vi "Kinect test.vi"() -> ()   [LabVIEW 2017]
uses:
  <vilib>/MakerHub/KinectOne/Private/Type Defs/HandLeftState.ctl
  <vilib>/MakerHub/KinectOne/Private/Initialize Image [Body Index].vi
  <vilib>/MakerHub/KinectOne/Private/Initialize Image [Depth].vi
  <vilib>/MakerHub/KinectOne/Private/Initialize Image [Color].vi
  <vilib>/MakerHub/KinectOne/Private/kinectRead [BodyIndexFrame].vi
  <vilib>/MakerHub/KinectOne/Private/kinectRead [DepthFrame].vi
  <vilib>/MakerHub/KinectOne/Private/kinectRead [BodyFrame].vi
  <vilib>/MakerHub/KinectOne/KinectOne.lvlib
panel:
  out "Body Index Image 4":T1(plugin-control)
  out "Body Index Image 3":T1(plugin-control)
  out "Body Index Image 2":T1(plugin-control)
  in  "stop":bool
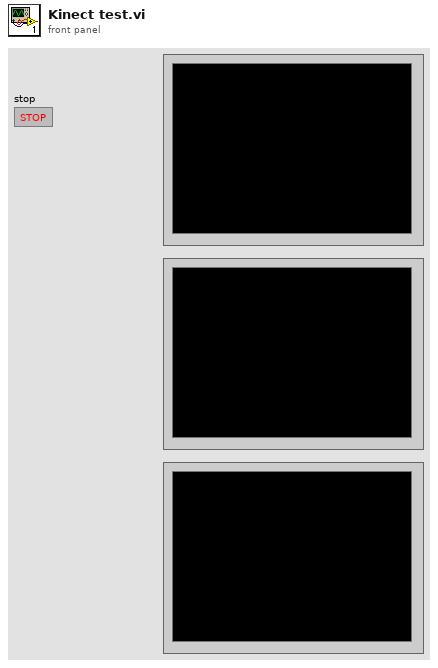
[diagram p1: front panel]
types:
  T1 = typedef "IMAQ Image.ctl" = refnum<image>
  T2 = typedef "KinectOne.lvlib/KinectSensor References.ctl" = cluster{"KinectSensor":refnum<k24>, "MultiSourceFrameReader":refnum<k24>, "BodyFrameDataInterface":refnum<k24>}
  T3 = typedef "KinectOne.lvlib/HandLeftState.ctl" = enum16{"Unknown", "NotTracked", "Open", "Closed", "Lasso"}
  T4 = typedef "KinectOne.lvlib/BodyData.ctl" = cluster{"ClippedEdges":T5, "HandLeftConfidence":T6, "HandLeftState":T3, "HandRightConfidence":T7, "HandRightState":T8, "IsRestricted":bool, "IsTracked":bool, "JointOrientations":refnum<k24>, "Joints":refnum<k24>, "Lean":refnum<k24>, "LeanTrackingState":T9, "TrackingId":u64}
  T5 = typedef "KinectOne.lvlib/ClippedEdges.ctl" = enum16{"None", "Right", "Left", "Top", "Bottom"}
  T6 = typedef "KinectOne.lvlib/HandLeftConfidence.ctl" = enum16{"Low", "High"}
  T7 = typedef "KinectOne.lvlib/HandRightConfidence.ctl" = enum16{"Low", "High"}
  T8 = typedef "KinectOne.lvlib/HandRightState.ctl" = enum16{"Unknown", "NotTracked", "Open", "Closed", "Lasso"}
  T9 = typedef "KinectOne.lvlib/LeanTrackingState.ctl" = enum16{"NotTracked", "Inferred", "Tracked"}
  T10 = cluster{"Body Data[0]":T4, "Body Data[1]":T4, "Body Data[2]":T4, "Body Data[3]":T4, "Body Data[4]":T4, "Body Data[5]":T4, "Body Data[6]":T4, "Body Data[7]":T4, "Body Data[8]":T4}
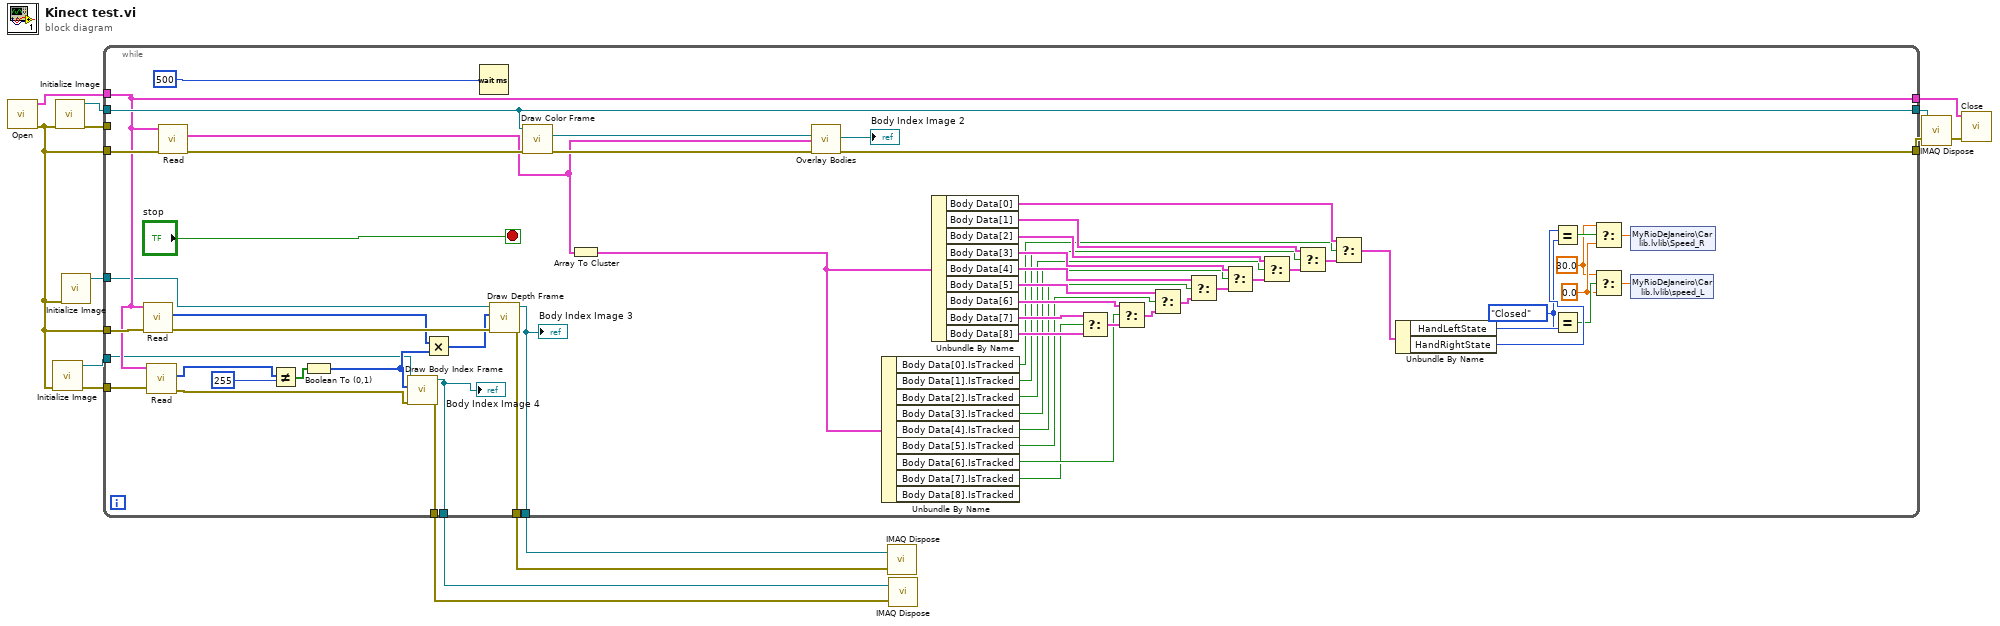
[diagram p0: block diagram]
diagram:
  n1 = call <vilib>:"Open.vi"() -> ("Error Out"=w5:errorcluster, "KinectSensor References out"=w13:T2)  [unwired: 10 in]
  n2 = call-poly <vilib>:"Initialize Image.vi"("Error In"=w5) -> ("Error Out"=w4:errorcluster, "Body Index Image"=w3:T1)  [unwired: 9 in]
  n3 = call-poly <vilib>:"Initialize Image.vi"("Error In"=w5) -> ("Error Out"=w12:errorcluster, "Color Image"=w14:T1)  [unwired: 9 in]
  n4 = call-poly <vilib>:"Initialize Image.vi"("Error In"=w5) -> ("Depth Image"=w8:T1)  [unwired: 9 in, 1 out]
  n5 = while {
    tunnel: w14 -> [w70]
    tunnel: w13 -> [w27]
    tunnel: w12 -> [_]
    tunnel: w5 -> [w74]
    tunnel: [w73] -> w11
    tunnel: [w70] -> w9
    tunnel: [w27] -> w10
    tunnel: w5 -> [w32]
    tunnel: w8 -> [w17]
    tunnel: [w30] -> w7
    tunnel: [w29] -> w6
    tunnel: w4 -> [w28]
    tunnel: w3 -> [w18]
    tunnel: [w24] -> w2
    tunnel: [w25] -> w1
    stop <- "stop" stop-if-true
    w35 = 30.0 ("f")
    w36 = 0.0 ("f")
    w39 = HandLeftState."Closed" ("y")
    n6 = call-poly <vilib>:"Read.vi"("Error In"=w32, "KinectSensor References in"=w27) -> ("Error Out"=w31:errorcluster, "frameData"=w20:u16[])  [unwired: 7 in, 1 out]
    n7 = call-poly <vilib>:"Read.vi"("Error In"=w28, "KinectSensor References in"=w27) -> ("Error Out"=w26:errorcluster, "frameData"=w23:u8[])  [unwired: 7 in, 1 out]
    n8 = call-poly <vilib>:"Read.vi"("error in (no error)"=w74, "KinectSensor References in"=w27) -> ("error out"=w69:errorcluster, "Body Data"=w68:T4[])  [unwired: 7 in, 1 out]
    n9 = Not Equal?(x=w23, y=255) -> (x != y?=w22:bool[])
    n10 = Boolean To (0,1)(Boolean=w22) -> (0, 1=w19:i16[])
    n11 = call <vilib>:"Draw Body Index Frame.vi"("Error In"=w26, "Byte Array"=w19, "Image"=w18) -> ("Error Out"=w25:errorcluster, "Image Out"=w24:T1)  [unwired: 7 in]
    "Body Index Image 4" <- w24
    n12 = Multiply(x=w20, y=w19) -> (x*y=w16:u16[])
    n13 = Wait (ms)(milliseconds to wait=u32 500) -> ()  [unwired: 1 out]
    n14 = call <vilib>:"Draw Depth Frame.vi"("Error In"=w31, "U16 Array"=w16, "Image"=w17) -> ("Error Out"=w30:errorcluster, "Image Out"=w29:T1)  [unwired: 7 in]
    "Body Index Image 3" <- w29
    n15 = call <vilib>:"Draw Color Frame.vi"("Error In"=w69, "Image"=w70) -> ("Error Out"=w71:errorcluster, "Image Out"=w72:T1)  [unwired: 8 in]
    n16 = Array To Cluster(array=w68) -> (cluster=w67:T10)
    n17 = call <vilib>:"Overlay Bodies.vi"("Error In"=w71, "Image"=w72, "Body Data"=w68) -> ("Error Out"=w73:errorcluster, "Image Out"=→"Body Index Image 2":T1)  [unwired: 7 in]
    n18 = Unbundle By Name(w67) -> ("Body Data[0].IsTracked"=w50:bool, "Body Data[1].IsTracked"=w49:bool, "Body Data[2].IsTracked"=w48:bool, "Body Data[3].IsTracked"=w47:bool, "Body Data[4].IsTracked"=w46:bool, "Body Data[5].IsTracked"=w45:bool, "Body Data[6].IsTracked"=w44:bool, "Body Data[7].IsTracked"=w43:bool)  [unwired: 1 out]
    n19 = Unbundle By Name(w67) -> ("Body Data[0]"=w63:T4, "Body Data[1]"=w54:T4, "Body Data[2]"=w55:T4, "Body Data[3]"=w56:T4, "Body Data[4]"=w58:T4, "Body Data[5]"=w59:T4, "Body Data[6]"=w60:T4, "Body Data[7]"=w65:T4, "Body Data[8]"=w66:T4)
    n20 = Select(t=w65, s=w43, f=w66) -> (s? t:f=w64:T4)
    n21 = Select(t=w60, s=w44, f=w64) -> (s? t:f=w62:T4)
    n22 = Select(t=w59, s=w45, f=w62) -> (s? t:f=w61:T4)
    n23 = Select(t=w58, s=w46, f=w61) -> (s? t:f=w57:T4)
    n24 = Select(t=w56, s=w47, f=w57) -> (s? t:f=w51:T4)
    n25 = Select(t=w55, s=w48, f=w51) -> (s? t:f=w52:T4)
    n26 = Select(t=w54, s=w49, f=w52) -> (s? t:f=w53:T4)
    n27 = Select(t=w63, s=w50, f=w53) -> (s? t:f=w42:T4)
    n28 = Unbundle By Name(w42) -> ("HandLeftState"=w41:T3, "HandRightState"=w40:T8)
    n29 = Equal?(x=w40, y=w39) -> (x = y?=w38:bool)
    n30 = Equal?(x=w41, y=w39) -> (x = y?=w37:bool)
    n31 = Select(t=w35, s=w38, f=w36) -> (s? t:f=w33:dbl)
    n32 = Select(t=w35, s=w37, f=w36) -> (s? t:f=w34:dbl)
    n33 = shared-variable "MyRioDeJaneiro\\Car lib.lvlib\\Speed_R"(w33) -> ()  [unwired: 1 in, 1 out]
    n34 = shared-variable "MyRioDeJaneiro\\Car lib.lvlib\\speed_L"(w34) -> ()  [unwired: 1 in, 1 out]
  }
  n35 = call "IMAQ Dispose"("Image"=w6, "error in (no error)"=w7) -> ()  [unwired: 4 in, 1 out]
  n36 = call "IMAQ Dispose"("Image"=w2, "error in (no error)"=w1) -> ()  [unwired: 4 in, 1 out]
  n37 = call "IMAQ Dispose"("Image"=w9, "error in (no error)"=w11) -> ("error out"=w15:errorcluster)  [unwired: 4 in]
  n38 = call <vilib>:"Close.vi"("Error In"=w15, "KinectSensor References"=w10) -> ()  [unwired: 9 in, 1 out]
